vi "Configure Tool Rack.vi"(8 "error in (no error)":errorcluster, 11 "WorkTable Class in":refnum<class "WorkTable Class.lvclass">) -> (0 "error out":errorcluster, 3 "WorkTable Class out":refnum<class "WorkTable Class.lvclass">)   [LabVIEW 2011, in "WorkTable Class.lvclass"]
uses:
  WorkTable Class.lvclass
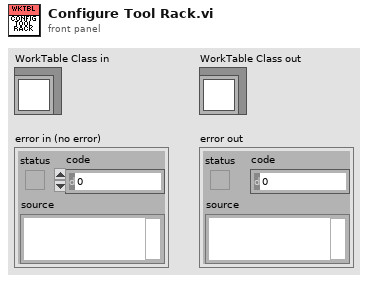
[diagram p1: front panel]
types:
  T1 = enum16{"None", "Grabber", "Picker", "Tool Setter"}
  T2 = cluster{"Position 1":enum16{"None", "Grabber", "Picker", "Tool Setter"}, "Position 2":enum16{"None", "Grabber", "Picker", "Tool Setter"}, "Position 3":enum16{"None", "Grabber", "Picker", "Tool Setter"}}
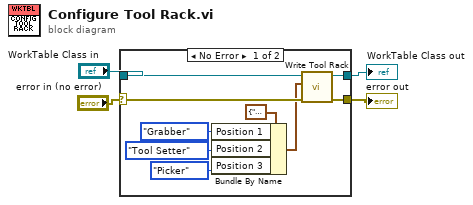
[diagram p0: block diagram]
diagram:
  n1 = case shown="No Error" "error in (no error)" {
    selector: "error in (no error)" -> [w10 w15]
    tunnel: [w12 w15] -> w1
    tunnel: [w13 w14] -> w2
    tunnel: "WorkTable Class in" -> [w11 w14]
    frame No Error {
      n2 = Bundle By Name(cluster=T2 {"Position 1"=enum."None", "Position 2"=enum."None", "Position 3"=enum."None"} ("Tool Rack"), "Position 1"=T1."Grabber", "Position 2"=T1."Tool Setter", "Position 3"=T1."Picker") -> (w5:T2)
      n3 = call-dynamic "Write Tool Rack.vi"("error in (no error)"=w10, "Tool Rack"=w5, "WorkTable Class in"=w11) -> ("error out"=w12:errorcluster, "WorkTable Class out"=w13:refnum<class "WorkTable Class.lvclass">)  [unwired: 7 in]
    }
    frame Error {
    }
  }
  "WorkTable Class out" <- w2
  "error out" <- w1
